vi "GetBarHeight.vi"(8 "error in (no error)":errorcluster, 11 "BarCode in":refnum<class "Linear Barcode.lvclass">) -> (0 "error out":errorcluster, 2 "Bar Height":u8=15, 3 "BarCode out":refnum<class "Linear Barcode.lvclass">)   [LabVIEW 2013, in "BarCodes.lvlib" / "Linear Barcode.lvclass"]
doc: "Returns the height of the barcode. This is read only because it is generally set by the barcode specification."
uses:
  Linear Barcode/Linear Barcode.lvclass
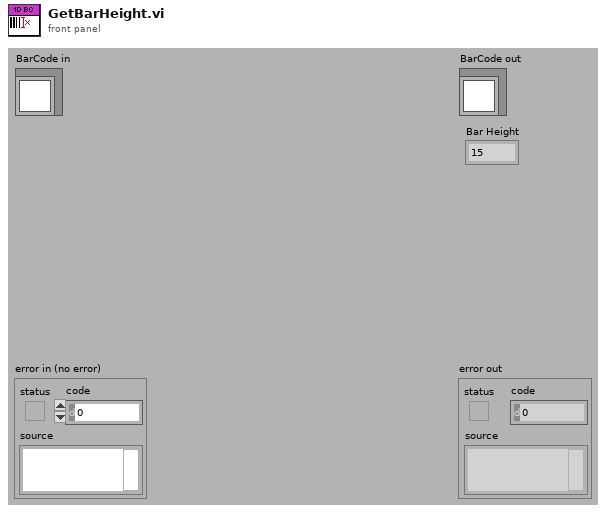
[diagram p1: front panel]
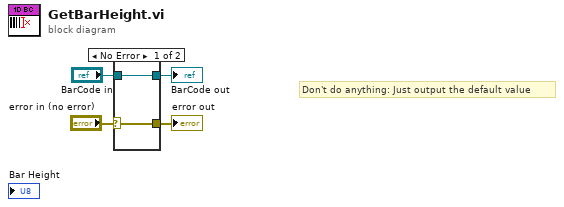
[diagram p0: block diagram]
diagram:
  # "Don't do anything: Just output the default value"
  n1 = case shown="No Error" "error in (no error)" {
    selector: "error in (no error)" -> [w5 w8]
    tunnel: [w5 w8] -> w3
    tunnel: [w6 w7] -> w1
    tunnel: "BarCode in" -> [w6 w7]
    frame No Error {
    }
    frame Error {
    }
  }
  "error out" <- w3
  "BarCode out" <- w1
